vi "Basic Test.vi"() -> ()   [LabVIEW 2016]
uses:
  <userlib>/_MGI/User Interface/Progress Bar/Progress Bar.lvclass
  <userlib>/_MGI/User Interface/Progress Bar/Progress Bar Settings/Progress Bar Settings.lvclass
panel:
  in  "Show on Taskbar":bool
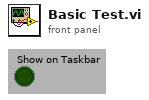
[diagram p1: front panel]
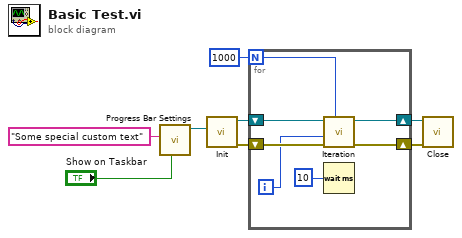
[diagram p0: block diagram]
diagram:
  n1 = call <userlib>:"Progress Bar Settings.vi"("Show on Taskbar (Win7 Only) (f)"="Show on Taskbar", "Window Title (Progress)"="Some special custom text") -> ("MGI_Progress Bar Settings"=w4:refnum<class "Progress Bar Settings.lvclass">)  [unwired: 9 in]
  n2 = call <userlib>:"Init.vi"("Settings"=w4) -> ("error out"=w7:errorcluster, "Progress Bar"=w1:refnum<data-value>)  [unwired: 9 in]
  n3 = for {
    N: 1000 -> [w10]
    shift-right: [w14] -> w8
    shift-left: w1 -> [w15]
    shift-right: [w12] -> w6
    shift-left: w7 -> [w13]
    i -> [w9]
    n4 = call <userlib>:"Iteration.vi"("Total Iterations"=w10, "error in (no error)"=w13, "Current Iteration"=w9, "Progress Bar"=w15) -> ("error out"=w12:errorcluster, "Progress Bar"=w14:refnum<data-value>)  [unwired: 5 in, 1 out]
    n5 = Wait (ms)(milliseconds to wait=u32 10) -> ()  [unwired: 1 out]
  }
  n6 = call <userlib>:"Close.vi"("error in (no error)"=w6, "Progress Bar"=w8) -> ()  [unwired: 9 in, 1 out]
